vi "Actor Core.vi"(8 "error in":errorcluster, 11 "EmulatorActor in":refnum<class "EmulatorActor.lvclass">) -> (0 "error out":errorcluster, 3 "Actor out":refnum<class "Actor.lvclass">)   [LabVIEW 2019, in "EmulatorActor.lvlib" / "EmulatorActor.lvclass"]
doc: "(<B>Filename</B>: Actor Framework.lvlib:Actor.lvclass:Actor Core.vi)\n\nReceives messages to the actor, reacts to them, and initiates any error handling that may shut the actor down.\n\nDescendant classes may override this VI to append parallel tasks for the actor to complete while it handles messages. Overrides use the Call Parent Method node."
uses:
  EmulatorActor.lvclass
  C:/Program Files (x86)/National Instruments/LabVIEW 2019/vi.lib/ActorFramework/Actor/Actor.lvclass
  <vilib>/ActorFramework/Actor/Actor.lvclass
  <vilib>/ActorFramework/Actor/Actor.lvclass/Actor.ctl
  <vilib>/ActorFramework/Message Enqueuer/Message Enqueuer.lvclass/Message Enqueuer.ctl
  EmulatorActor Messages/Generate Pulse Msg/Generate Pulse Msg.lvclass/Generate Pulse Msg.ctl
  <vilib>/ActorFramework/Message Enqueuer/Init from Existing Queue.vi
  <vilib>/ActorFramework/Message Enqueuer/Enqueue.vi
  EmulatorActor Messages/Generate Pulse Msg/Generate Pulse Msg.lvclass
  C:/Program Files (x86)/National Instruments/LabVIEW 2019/vi.lib/ActorFramework/Message/Message.lvclass
  <vilib>/ActorFramework/Stop Msg/Stop Msg.lvclass
  <vilib>/ActorFramework/Message Priority Queue/Priority Enqueue.vi
  <vilib>/ActorFramework/Message Enqueuer/Message Enqueuer.lvclass
panel:
  in  "Noise":dbl(knob) scale=0.0..10.0
  in  "Generate Pulse":bool
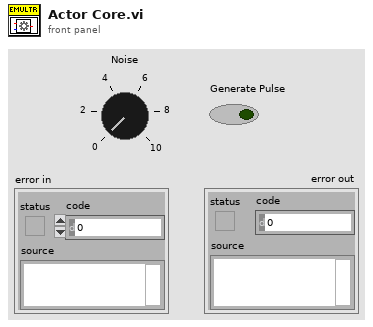
[diagram p1: front panel]
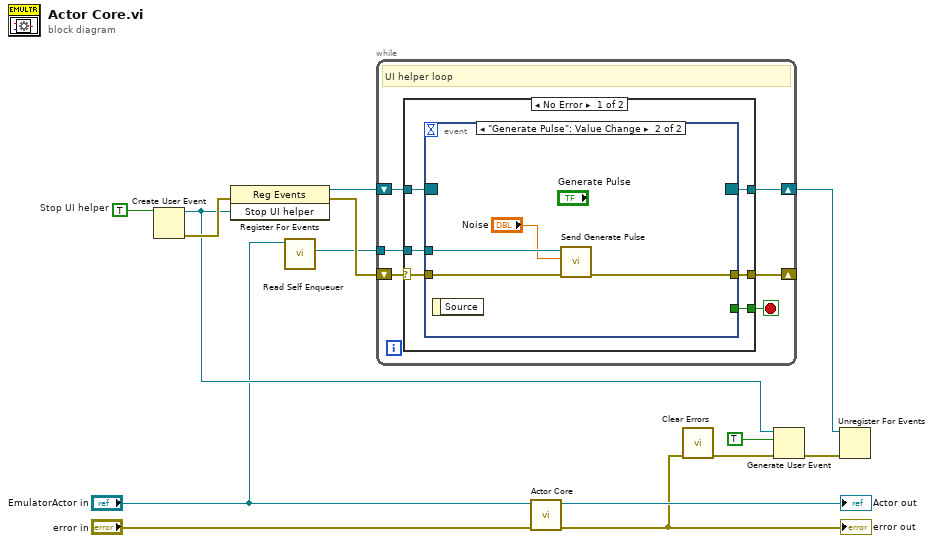
[diagram p0: block diagram]
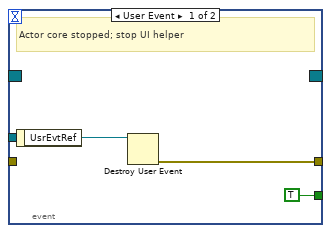
[diagram p2: hidden frame]
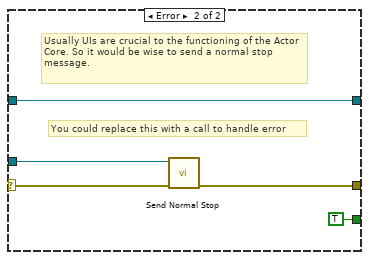
[diagram p3: hidden frame]
diagram:
  w11 = TRUE  # Stop UI helper
  n1 = Create User Event(user event datatype=w11) -> (user event=w7:refnum<user-event>, error out=w10:errorcluster)  [unwired: 1 in]
  n2 = register-events(error in=w10, w7) -> (reference out=w12:refnum<event-registration>, error out=w4:errorcluster)  [unwired: 1 in]
  n3 = call <vilib>:"Read Self Enqueuer.vi"("Actor"="EmulatorActor in") -> ("Self Enqueuer"=w3:refnum<class "Message Enqueuer.lvclass">)  [unwired: 10 in]
  n4 = while {
    shift-right: [w19] -> w9
    shift-left: w12 -> [w20]
    shift-right: [w16] -> _
    shift-left: w4 -> [w17]
    tunnel: w3 -> [w15]
    stop <- w18 stop-if-true
    # "UI helper loop"
    n5 = case shown="No Error" w17 {
      selector: w17 -> [w23 w36]
      tunnel: w20 -> [w26 w38]
      tunnel: [w25 w38] -> w19
      tunnel: [w24 TRUE] -> w18
      tunnel: [w22 w35] -> w16
      tunnel: w15 -> [w21 w34]
      frame No Error {
        n6 = event shown="[1] \"Generate Pulse\": Value Change" {
          selector: w26 -> [_ _]
          dyn-events: [_ _] -> w25
          timeout: _ -> [_ _]
          tunnel: [TRUE _] -> w24
          tunnel: w23 -> [_ w32]
          tunnel: [w27 w31] -> w22
          tunnel: w21 -> [_ w33]
          event User Event {
            # "Actor core stopped; stop UI helper"
            n7 = event-data() -> ("UsrEvtRef"=w28:refnum<user-event>)  [unwired: 1 in]
            n8 = Destroy User Event(user event=w28) -> (error out=w27:errorcluster)  [unwired: 1 in]
          }
          event "Generate Pulse": Value Change {
            n9 = event-data() -> ()  [unwired: 1 in, 1 out]
            n10 = call "Send Generate Pulse.vi"("error in (no error)"=w32, "Noise"="Noise", "Message Enqueuer"=w33) -> ("error out"=w31:errorcluster)  [unwired: 7 in, 1 out]
          }
        }
      }
      frame Error {
        # "You could replace this with a call to handle error"
        # "Usually UIs are crucial to the functioning of the Actor Core. So it would be wise to send a normal stop message."
        n11 = call <vilib>:"Send Normal Stop.vi"("error in (no error)"=w36, "Message Enqueuer"=w34) -> ("error out"=w35:errorcluster)  [unwired: 9 in]
      }
    }
  }
  n12 = call-parent "Actor Core.vi"("error in"="error in", "Actor in"="EmulatorActor in") -> ("error out"=w1:errorcluster, "Actor out"=→"Actor out":refnum<class "Actor.lvclass">)  [unwired: 8 in]
  "error out" <- w1
  n13 = call <vilib>:"Clear Errors.vi"("error in (no error)"=w1) -> ("error out"=w5:errorcluster)  [unwired: 5 in, 1 out]
  n14 = Generate User Event(user event=w7, event data cluster=TRUE ("event data"), error in=w5) -> (error out=w8:errorcluster)  [unwired: 1 in, 1 out]
  n15 = Unregister For Events(event registration refnum=w9, error in=w8) -> ()  [unwired: 1 out]
